vi "電磁.vi"() -> ()   [LabVIEW 2021]
uses:
  XControl 1.xctl
panel:
  out "XControl 1":bool(xcontrol)
  in  "Boolean":bool
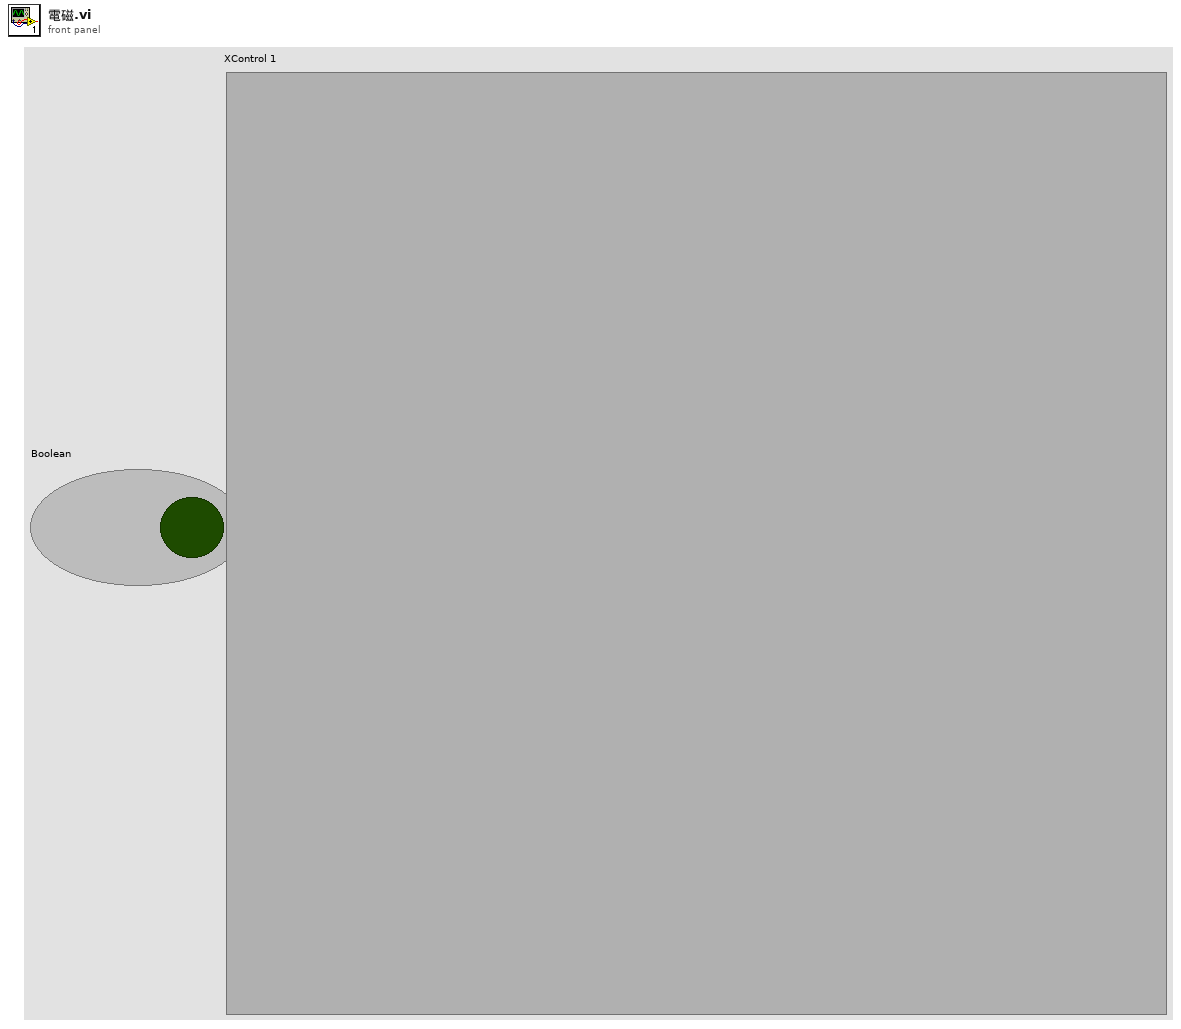
[diagram p1: front panel]
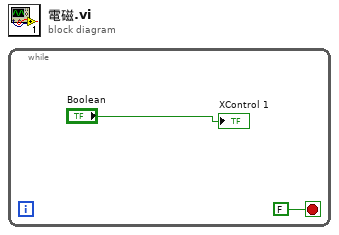
[diagram p0: block diagram]
diagram:
  n1 = while {
    stop <- FALSE stop-if-true
    "XControl 1" <- "Boolean"
  }
